vi "Lift.vi"(0 "LiftLocation":T1(ring)) -> ()   [LabVIEW 2018]
uses:
  <vilib>/Rock Robotics/SystemInterfaces/DIO/FPGA_DIOChannel.ctl
  <vilib>/Rock Robotics/WPI/ThirdParty/Phoenix-LabVIEW/Motor Controller/Controls/CTRE_Phoenix_MotorControl_ControlMode.ctl
  Lift Global.vi
  Times/Times Global.vi
  <vilib>/addons/control/pid/pid.llb/PID (DBL).vi
  <vilib>/Rock Robotics/WPI/ThirdParty/Phoenix-LabVIEW/Motor Controller/Get/CTRE_Phoenix_MotorController_GetSelectedSensorData.vi
  Cargo Intake/Cargo Intake Global.vi
  <vilib>/addons/control/pid/NI_PID_pid.lvlib
  <vilib>/Rock Robotics/WPI/Counter/WPI_CounterDigitalInputToDigitalSource.vi
panel:
  in  "t":dbl=0.5 format="%#_13g"
  in  "output range":cluster{"output high":dbl, "output low":dbl}={"output high"=1.0, "output low"=-1.0}
  in  "LiftMode":T2(ring)=enum."Basic Control"
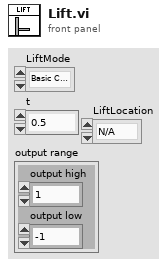
[diagram p1: front panel]
types:
  T1 = enum16{"N/A", "Hatch Panel Zone 1", "Hatch Panel Zone 2", "Hatch Panel Zone 3", "Cargo Zone 1", "Cargo Zone 2", "Cargo Zone 3"}
  T2 = enum16{"Ultra Manual Control", "Manual Control", "Basic Control", "Automated Control", "Autonomous Control"}
  T3 = typedef "FPGA_DIOChannel.ctl" = enum8{"DIO 0", "DIO 1", "DIO 2", "DIO 3", "DIO 4", "DIO 5", "DIO 6", "DIO 7", "DIO 8", "DIO 9", "DIO MXP 0", "DIO MXP 1", "DIO MXP 2", "DIO MXP 3", "DIO MXP 4", "DIO MXP 5", "DIO MXP 6", "DIO MXP 7", "DIO MXP 8", "DIO MXP 9", "DIO MXP 10", "DIO MXP 11", "DIO MXP 12", "DIO MXP 13", "DIO MXP 14", "DIO MXP 15", "SPI Port CS1", "SPI Port CS2", "SPI Port CS3", "SPI Port MISO", "SPI Port MOSI", "Invalid"}
  T4 = typedef "WPI_DigitalInputDevRef.ctl" = cluster{"DevStatus":errorcluster, "DIO Channel":T3}
  T5 = typedef "FPGA_CounterEncoderSourceConvertionLVSourceType.ctl" = cluster{"DevStatus":errorcluster, "AnalogTriggerMode?":bool, "DigitalMode":cluster{"DIO Channel":T6}, "AnalogTriggerMode":cluster{"AnalogTriggerIndex":T7, "OutputType":T8}}
  T6 = typedef "FPGA_DIODigitalSourceChannel.ctl" = enum8{"DIO 0", "DIO 1", "DIO 2", "DIO 3", "DIO 4", "DIO 5", "DIO 6", "DIO 7", "DIO 8", "DIO 9", "DIO MXP 0", "DIO MXP 1", "DIO MXP 2", "DIO MXP 3", "DIO MXP 4", "DIO MXP 5", "DIO MXP 6", "DIO MXP 7", "DIO MXP 8", "DIO MXP 9", "DIO MXP 10", "DIO MXP 11", "DIO MXP 12", "DIO MXP 13", "DIO MXP 14", "DIO MXP 15", "SPI Port CS1", "SPI Port CS2", "SPI Port CS3", "SPI Port MISO", "SPI Port MOSI", "Disabled"}
  T7 = typedef "FPGA_AnalogTriggerIndex.ctl" = enum8{"Trig 0", "Trig 1", "Trig 2", "Trig 3", "Trig 4", "Trig 5", "Trig 6", "Trig 7", "Invalid"}
  T8 = typedef "FPGA_AnalogTriggerOutType.ctl" = enum16{"InWindow", "TriggerState", "Rising", "Falling"}
  T9 = typedef "WPI_EncoderDevRef.ctl" = cluster{"DevStatus":errorcluster, "EncoderIndex":T10, "CounterIndex":T11, "DistancePerCount":dbl, "Decoding Type":T12}
  T10 = typedef "FPGA_EncoderIdx.ctl" = enum8{"Enc 0", "Enc 1", "Enc 2", "Enc 3", "Enc 4", "Enc 5", "Enc 6", "Enc 7", "Invalid"}
  T11 = typedef "FPGA_CounterCtrSystemIndex.ctl" = enum8{"Ctr 0", "Ctr 1", "Ctr 2", "Ctr 3", "Ctr 4", "Ctr 5", "Ctr 6", "Ctr 7", "Invalid"}
  T12 = typedef "WPI_EncoderType.ctl" = enum16{"1x", "2x", "4x"}
  T13 = typedef "WPI_MotorControlDeviceRef.ctl" = cluster{"DeviceStatus":errorcluster, "Type":T14, "PWM":cluster{"PWM Channel":T15, "DeadBand":T16}, "CAN":cluster{"Device Number":u8, "SetOutput VI Ref":variant, "GetOutput VI Ref":variant, "Enable VI Ref":variant, "Disable VI Ref":variant, "Data":variant}, "Invert":bool, "DIO PWM":cluster{"PWM \"Enable\" Channel":T15, "DIOChannel":T3, "PWM Rate":dbl}}
  T14 = typedef "WPI_MotorControlType.ctl" = enum16{"PWM", "CAN", "DIO PWM"}
  T15 = typedef "FPGA_DIOPWMChannel.ctl" = enum8{"PWM 0", "PWM 1", "PWM 2", "PWM 3", "PWM 4", "PWM 5", "PWM 6", "PWM 7", "PWM 8", "PWM 9", "PWM MXP 0", "PWM MXP 1", "PWM MXP 2", "PWM MXP 3", "PWM MXP 4", "PWM MXP 5", "PWM MXP 6", "PWM MXP 7", "PWM MXP 8", "PWM MXP 9", "Invalid"}
  T16 = typedef "WPI_PWMDeadband.ctl" = cluster{"Name":string, "maxPositivePwm":i32, "minPositivePwm":i32, "centerPwm":i32, "maxNegativePwm":i32, "minNegativePwm":i32, "angularRange":u16}
  T17 = typedef "CTRE_Phoenix_MotorControl_ControlMode.ctl" = u16
  T18 = typedef "Control 3.ctl" = dbl
  T19 = cluster{"proportional gain (Kc)":dbl, "integral time(Ti, min)":dbl, "derivative time(Td, min) 2":dbl}
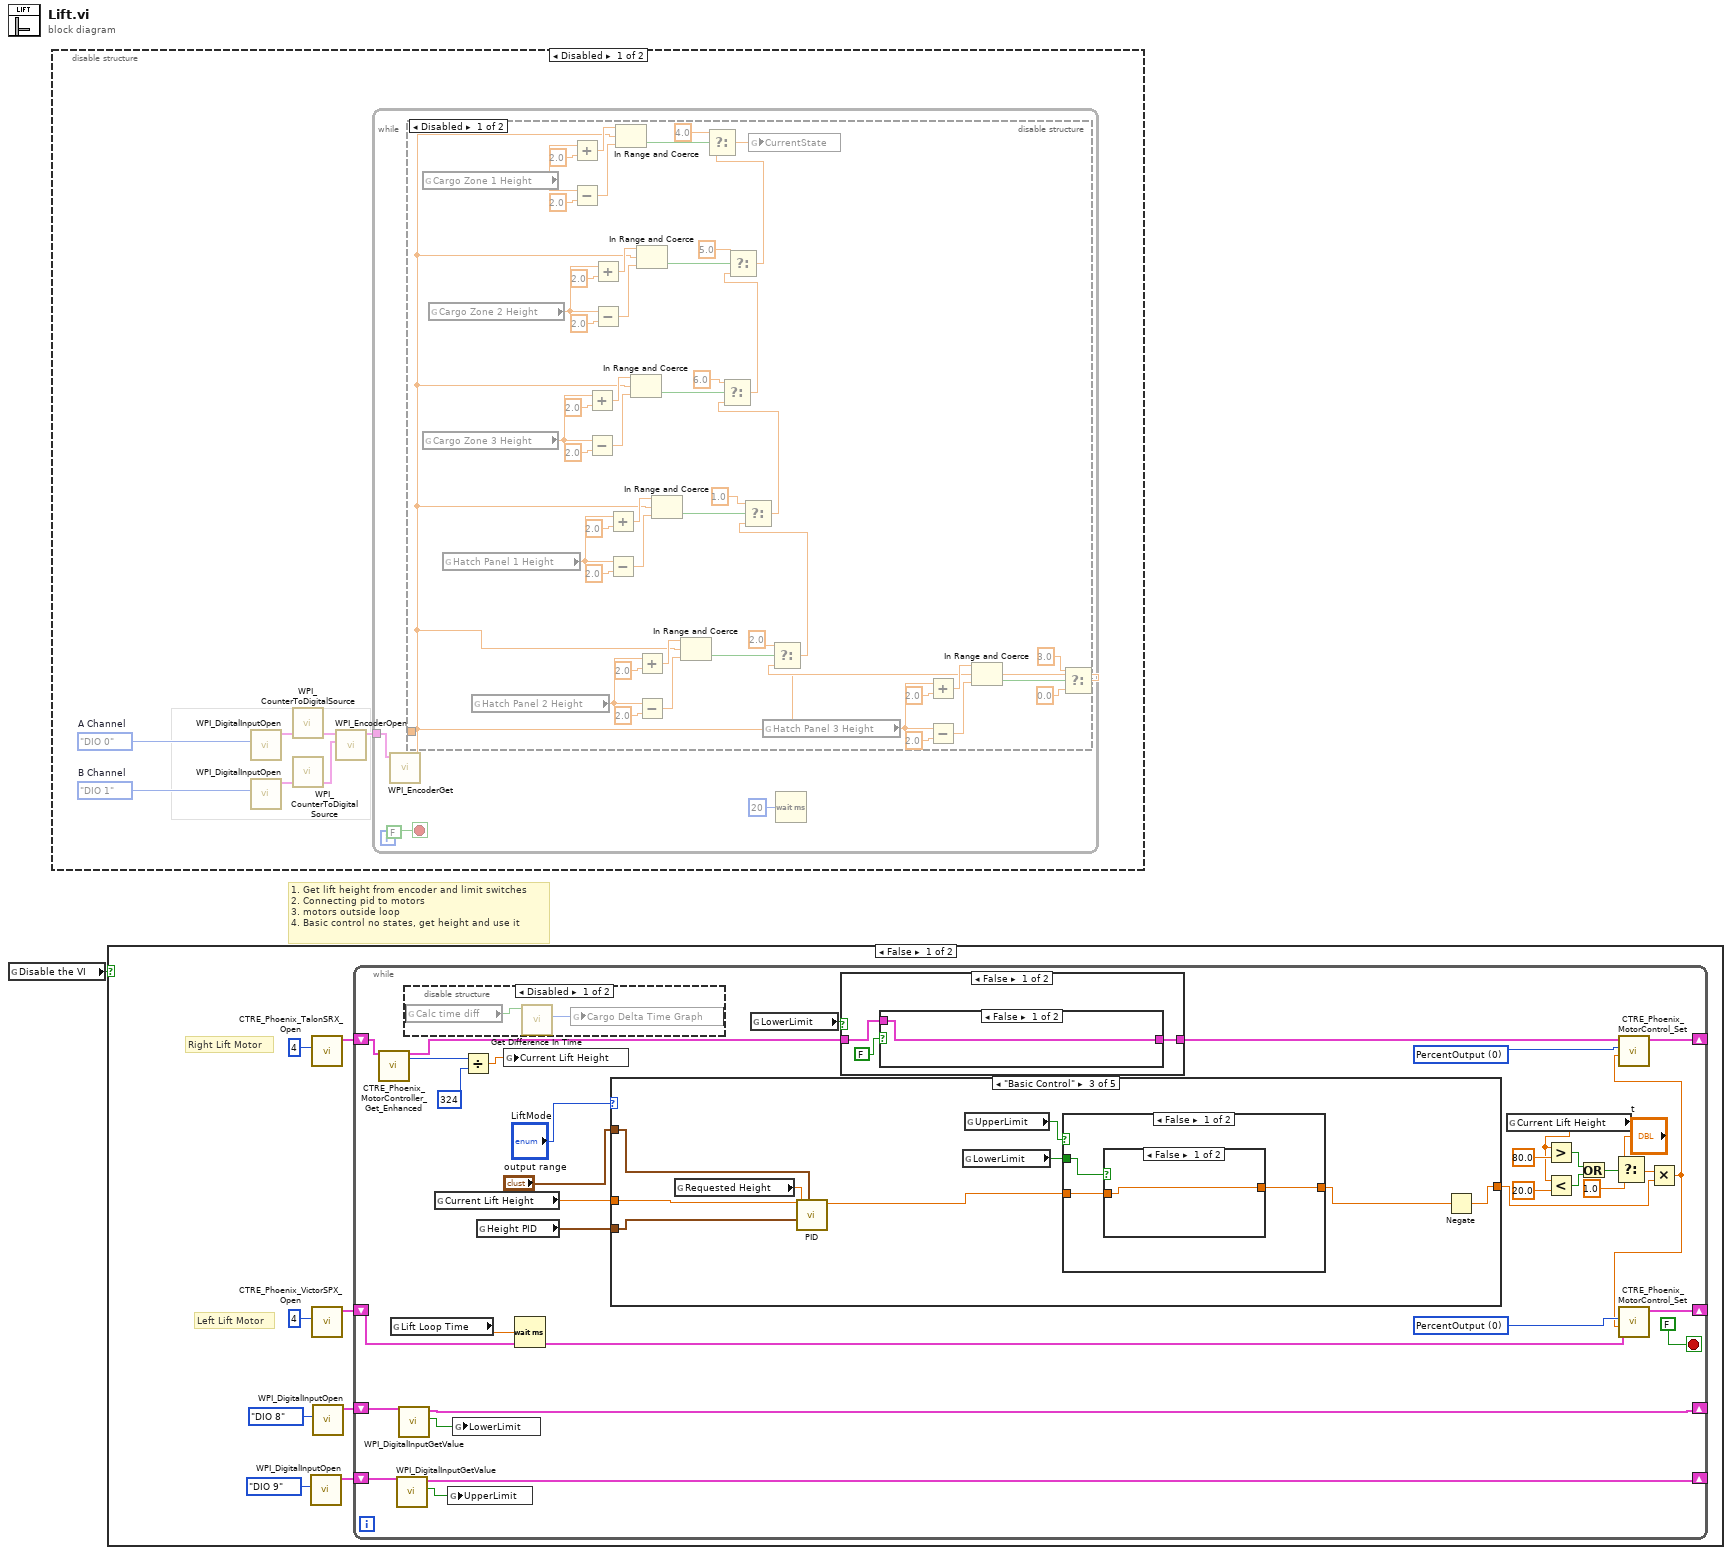
[diagram p0: block diagram]
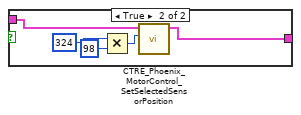
[diagram p4: hidden frame]
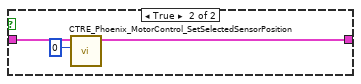
[diagram p5: hidden frame]
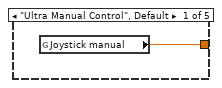
[diagram p7: hidden frame]
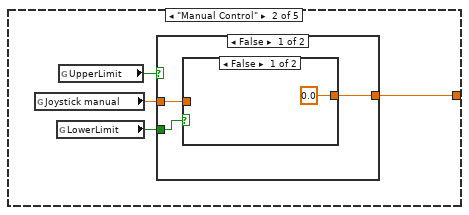
[diagram p8: hidden frame]
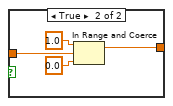
[diagram p9: hidden frame]
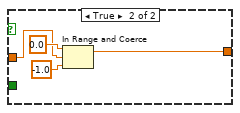
[diagram p10: hidden frame]
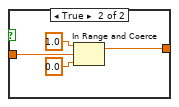
[diagram p11: hidden frame]
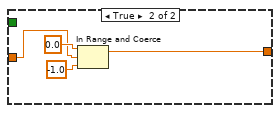
[diagram p12: hidden frame]
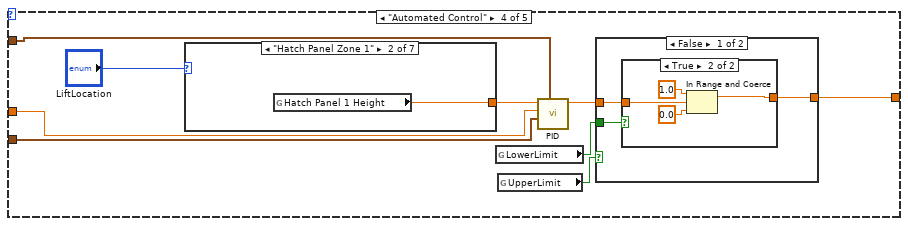
[diagram p13: hidden frame]
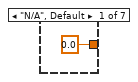
[diagram p14: hidden frame]
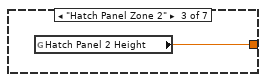
[diagram p15: hidden frame]
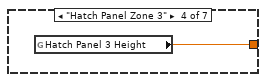
[diagram p16: hidden frame]
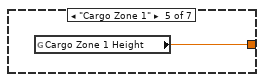
[diagram p17: hidden frame]
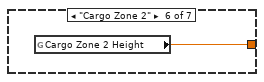
[diagram p18: hidden frame]
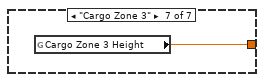
[diagram p19: hidden frame]
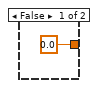
[diagram p20: hidden frame]
diagram:
  # "1. Get lift height from encoder and limit switches\n2. Connecting pid to motors\n3. motors outside loop\n4. Basic control no states, get height and use it"
  n1 = global read "Lift Global.vi" "Disable the VI"() -> (w1:bool)
  n2 = disable-structure shown="Disabled" {
    frame Disabled {
      w8 = FPGA_DIOChannel."DIO 1"  # B Channel
      w7 = FPGA_DIOChannel."DIO 0"  # A Channel
      n3 = call <vilib>:"WPI_DigitalInputOpen.vi"("DIO Channel"=w7) -> ("DigitalInputDevRef"=w4:T4)  [unwired: 1 in, 9 out]
      n4 = call <vilib>:"WPI_DigitalInputOpen.vi"("DIO Channel"=w8) -> ("DigitalInputDevRef"=w5:T4)  [unwired: 1 in, 9 out]
      n5 = call-poly <vilib>:"WPI_CounterToDigitalSource.vi"("DigitalInputDevRef"=w4) -> ("Digital Source"=w3:T5)  [unwired: 6 out]
      n6 = call-poly <vilib>:"WPI_CounterToDigitalSource.vi"("DigitalInputDevRef"=w5) -> ("Digital Source"=w6:T5)  [unwired: 6 out]
      n7 = call <vilib>:"WPI_EncoderOpen.vi"("BSource"=w6, "ASource"=w3) -> ("EncoderDevRef"=w2:T9)  [unwired: 6 in, 3 out]
      n8 = while {
        tunnel: w2 -> [w12]
        stop <- FALSE stop-if-true
        n9 = call <vilib>:"WPI_EncoderGet.vi"("EncoderDevRef"=w12) -> ("Distance"=w10:dbl)  [unwired: 5 in, 5 out]
        n10 = disable-structure shown="Disabled" {
          disable-tunnel: w10 -> [w13 _]
          frame Disabled {
            n11 = global read "Lift Global.vi" "Cargo Zone 1 Height"() -> (w53:dbl)
            n12 = global read "Lift Global.vi" "Cargo Zone 3 Height"() -> (w41:dbl)
            n13 = global read "Lift Global.vi" "Cargo Zone 2 Height"() -> (w59:dbl)
            n14 = global read "Lift Global.vi" "Hatch Panel 1 Height"() -> (w47:dbl)
            n15 = global read "Lift Global.vi" "Hatch Panel 2 Height"() -> (w29:dbl)
            n16 = Add(x=w53, y=2.0) -> (x+y=w55:dbl)
            n17 = Subtract(x=w53, y=2.0) -> (x-y=w56:dbl)
            n18 = Add(x=w41, y=2.0) -> (x+y=w43:dbl)
            n19 = Subtract(x=w41, y=2.0) -> (x-y=w44:dbl)
            n20 = Add(x=w59, y=2.0) -> (x+y=w61:dbl)
            n21 = Subtract(x=w59, y=2.0) -> (x-y=w62:dbl)
            n22 = Add(x=w47, y=2.0) -> (x+y=w49:dbl)
            n23 = Subtract(x=w47, y=2.0) -> (x-y=w50:dbl)
            n24 = In Range and Coerce(upper limit=w55, x=w13, lower limit=w56) -> (In Range?=w51:bool)  [unwired: 1 out]
            n25 = In Range and Coerce(upper limit=w43, x=w13, lower limit=w44) -> (In Range?=w39:bool)  [unwired: 1 out]
            n26 = In Range and Coerce(upper limit=w61, x=w13, lower limit=w62) -> (In Range?=w57:bool)  [unwired: 1 out]
            n27 = Add(x=w29, y=2.0) -> (x+y=w31:dbl)
            n28 = Subtract(x=w29, y=2.0) -> (x-y=w32:dbl)
            n29 = In Range and Coerce(upper limit=w49, x=w13, lower limit=w50) -> (In Range?=w45:bool)  [unwired: 1 out]
            n30 = In Range and Coerce(upper limit=w31, x=w13, lower limit=w32) -> (In Range?=w27:bool)  [unwired: 1 out]
            n31 = global read "Lift Global.vi" "Hatch Panel 3 Height"() -> (w35:dbl)
            n32 = Add(x=w35, y=2.0) -> (x+y=w37:dbl)
            n33 = Subtract(x=w35, y=2.0) -> (x-y=w38:dbl)
            n34 = In Range and Coerce(upper limit=w37, x=w13, lower limit=w38) -> (In Range?=w33:bool)  [unwired: 1 out]
            n35 = Select(t=3.0, s=w33, f=0.0 ("t")) -> (s? t:f=w23:dbl)
            n36 = Select(t=2.0, s=w27, f=w23) -> (s? t:f=w24:dbl)
            n37 = Select(t=1.0, s=w45, f=w24) -> (s? t:f=w25:dbl)
            n38 = Select(t=6.0, s=w39, f=w25) -> (s? t:f=w26:dbl)
            n39 = Select(t=5.0, s=w57, f=w26) -> (s? t:f=w20:dbl)
            n40 = Select(t=4.0, s=w51, f=w20) -> (s? t:f=w21:dbl)
            n41 = global write "Lift Global.vi" "CurrentState"(w21) -> ()
          }
          frame Enabled {
          }
        }
        n42 = Wait (ms)(milliseconds to wait=u32 20) -> ()  [unwired: 1 out]
      }
    }
    frame Enabled {
    }
  }
  n43 = case shown="False" w1 {
    frame False {
      # "Left Lift Motor"
      # "Right Lift Motor"
      n44 = call <vilib>:"WPI_DigitalInputOpen.vi"("DIO Channel"=FPGA_DIOChannel."DIO 9") -> ("DigitalInputDevRef"=w63:T4)  [unwired: 9 in, 1 out]
      n45 = call <vilib>:"CTRE_Phoenix_TalonSRX_Open.vi"("Device Number"=u8 4) -> ("CAN Talon SRX Ref"=w70:T13)  [unwired: 9 in, 1 out]
      n46 = call <vilib>:"CTRE_Phoenix_VictorSPX_Open.vi"("Device Number"=u8 4) -> ("CAN Talon SRX Ref"=w68:T13)  [unwired: 9 in, 1 out]
      n47 = call <vilib>:"WPI_DigitalInputOpen.vi"("DIO Channel"=FPGA_DIOChannel."DIO 8") -> ("DigitalInputDevRef"=w65:T4)  [unwired: 9 in, 1 out]
      n48 = while {
        shift-right: [w101] -> _
        shift-left: w70 -> [w94]
        shift-right: [w99] -> _
        shift-left: w68 -> [w98]
        shift-right: [w87] -> _
        shift-left: w65 -> [w88]
        shift-right: [w82] -> _
        shift-left: w63 -> [w83]
        stop <- FALSE stop-if-true
        w100 = T17 0 items=["PercentOutput"=0, "Position"=1, "Velocity"=2, "Current"=3, "Follower"=5, "MotionProfile"=6, "MotionMagic"=7, "MotionProfileArc"=10, "Disabled"=15] ("Control Mode")
        w102 = T17 0 items=["PercentOutput"=0, "Position"=1, "Velocity"=2, "Current"=3, "Follower"=5, "MotionProfile"=6, "MotionMagic"=7, "MotionProfileArc"=10, "Disabled"=15] ("Control Mode")
        n49 = call-poly <vilib>:"CTRE_Phoenix_MotorController_Get_Enhanced.vi"("PhoenixMotorControlDevRef"=w94) -> ("PhoenixMotorControlDevRef"=w93:T13, "Position (Raw Sensor Units)"=w91:i32)  [unwired: 11 in, 2 out]
        n50 = global read "Times Global.vi" "Lift Loop Time"() -> (w105:T18)
        n51 = call <vilib>:"WPI_DigitalInputGetValue.vi"("DigitalInputDevRef"=w83) -> ("Value"=w85:bool, "DigitalInputDevRef"=w82:T4)  [unwired: 8 in, 1 out]
        n52 = call <vilib>:"WPI_DigitalInputGetValue.vi"("DigitalInputDevRef"=w88) -> ("Value"=w86:bool, "DigitalInputDevRef"=w87:T4)  [unwired: 8 in, 1 out]
        n53 = disable-structure shown="Disabled" {
          frame Disabled {
            n54 = global read "Cargo Intake Global.vi" "Calc time diff"() -> (w119:bool)
            n55 = call "Get Difference In Time.vi"("Calculate Time Difference"=w119) -> ("Delta Time over Time"=w118:u32)  [unwired: 9 in, 1 out]
            n56 = global write "Times Global.vi" "Cargo Delta Time Graph"(w118) -> ()
          }
          frame Enabled {
          }
        }
        n57 = global read "Lift Global.vi" "Current Lift Height"() -> (w95:dbl)
        n58 = global write "Lift Global.vi" "UpperLimit"(w85) -> ()
        n59 = global write "Lift Global.vi" "LowerLimit"(w86) -> ()
        n60 = Divide(x=w91, y=324) -> (x/y=w90:dbl)
        n61 = global read "Lift Global.vi" "Height PID"() -> (w96:T19)
        n62 = global write "Lift Global.vi" "Current Lift Height"(w90) -> ()
        n63 = Wait (ms)(milliseconds to wait=w105) -> ()  [unwired: 1 out]
        n64 = case shown="\"Basic Control\"" "LiftMode" {
          tunnel: [w120 w121 w141 w163 0.0 ("Cargo Zone 3 Height")] -> w74
          tunnel: w95 -> [_ _ w145 w161 _]
          tunnel: w96 -> [_ _ w144 w160 _]
          tunnel: "output range" -> [_ _ w143 w162 _]
          frame "Ultra Manual Control", Default {
            n65 = global read "Lift Global.vi" "Joystick manual"() -> (w120:dbl)
          }
          frame "Manual Control" {
            n66 = global read "Lift Global.vi" "Joystick manual"() -> (w122:dbl)
            n67 = global read "Lift Global.vi" "LowerLimit"() -> (w124:bool)
            n68 = global read "Lift Global.vi" "UpperLimit"() -> (w123:bool)
            n69 = case shown="False" w123 {
              tunnel: w124 -> [w127 _]
              tunnel: [w126 w134] -> w121
              tunnel: w122 -> [w125 w133]
              frame False {
                n70 = case shown="False" w127 {
                  tunnel: [0.0 w132] -> w126
                  tunnel: w125 -> [_ w129]
                  frame False {
                  }
                  frame True {
                    n71 = In Range and Coerce(upper limit=1.0, x=w129, lower limit=0.0) -> (coerced(x)=w132:dbl)  [unwired: 1 out]
                  }
                }
              }
              frame True {
                n72 = In Range and Coerce(upper limit=0.0, x=w133, lower limit=-1.0) -> (coerced(x)=w134:dbl)  [unwired: 1 out]
              }
            }
          }
          frame "Basic Control" {
            n73 = global read "Lift Global.vi" "Requested Height"() -> (w142:dbl)
            n74 = call-poly <vilib>:"PID.vi"("output range"=w143, "PID gains"=w144, "process variable"=w145, "setpoint"=w142) -> ("output"=w138:dbl)  [unwired: 6 in, 1 out]
            n75 = global read "Lift Global.vi" "LowerLimit"() -> (w140:bool)
            n76 = global read "Lift Global.vi" "UpperLimit"() -> (w139:bool)
            n77 = case shown="False" w139 {
              tunnel: w140 -> [w148 _]
              tunnel: [w147 w155] -> w137
              tunnel: w138 -> [w146 w154]
              frame False {
                n78 = case shown="False" w148 {
                  tunnel: [w149 w153] -> w147
                  tunnel: w146 -> [w149 w150]
                  frame False {
                  }
                  frame True {
                    n79 = In Range and Coerce(upper limit=1.0, x=w150, lower limit=0.0) -> (coerced(x)=w153:dbl)  [unwired: 1 out]
                  }
                }
              }
              frame True {
                n80 = In Range and Coerce(upper limit=0.0, x=w154, lower limit=-1.0) -> (coerced(x)=w155:dbl)  [unwired: 1 out]
              }
            }
            n81 = Negate(x=w137) -> (-x=w141:dbl)
          }
          frame "Automated Control" {
            n82 = case shown="\"Hatch Panel Zone 1\"" "LiftLocation" {
              tunnel: [0.0 ("Cargo Zone 3 Height") w168 w169 w170 w171 w172 w173] -> w158
              frame "N/A", Default {
              }
              frame "Hatch Panel Zone 1" {
                n83 = global read "Lift Global.vi" "Hatch Panel 1 Height"() -> (w168:dbl)
              }
              frame "Hatch Panel Zone 2" {
                n84 = global read "Lift Global.vi" "Hatch Panel 2 Height"() -> (w169:dbl)
              }
              frame "Hatch Panel Zone 3" {
                n85 = global read "Lift Global.vi" "Hatch Panel 3 Height"() -> (w170:dbl)
              }
              frame "Cargo Zone 1" {
                n86 = global read "Lift Global.vi" "Cargo Zone 1 Height"() -> (w171:dbl)
              }
              frame "Cargo Zone 2" {
                n87 = global read "Lift Global.vi" "Cargo Zone 2 Height"() -> (w172:dbl)
              }
              frame "Cargo Zone 3" {
                n88 = global read "Lift Global.vi" "Cargo Zone 3 Height"() -> (w173:dbl)
              }
            }
            n89 = global read "Lift Global.vi" "LowerLimit"() -> (w166:bool)
            n90 = global read "Lift Global.vi" "UpperLimit"() -> (w165:bool)
            n91 = call-poly <vilib>:"PID.vi"("output range"=w162, "PID gains"=w160, "process variable"=w161, "setpoint"=w158) -> ("output"=w164:dbl)  [unwired: 6 in, 1 out]
            n92 = case shown="False" w165 {
              tunnel: w166 -> [w176 _]
              tunnel: [w175 w183] -> w163
              tunnel: w164 -> [w174 w182]
              frame False {
                n93 = case shown="True" w176 {
                  tunnel: [0.0 w181] -> w175
                  tunnel: w174 -> [_ w178]
                  frame False {
                  }
                  frame True {
                    n94 = In Range and Coerce(upper limit=1.0, x=w178, lower limit=0.0) -> (coerced(x)=w181:dbl)  [unwired: 1 out]
                  }
                }
              }
              frame True {
                n95 = In Range and Coerce(upper limit=0.0, x=w182, lower limit=-1.0) -> (coerced(x)=w183:dbl)  [unwired: 1 out]
              }
            }
          }
          frame "Autonomous Control" {
          }
        }
        n96 = global read "Lift Global.vi" "LowerLimit"() -> (w84:bool)
        n97 = case shown="False" w84 {
          tunnel: w93 -> [w108 w117]
          tunnel: [w107 w116] -> w92
          frame False {
            n98 = case shown="False" FALSE {
              tunnel: w108 -> [w109 w114]
              tunnel: [w109 w113] -> w107
              frame False {
              }
              frame True {
                n99 = Multiply(x=324 ("y"), y=98 ("New Sensor Position")) -> (x*y=w110:i32)
                n100 = call <vilib>:"CTRE_Phoenix_MotorControl_SetSelectedSensorPosition.vi"("New Sensor Position"=w110, "PhoenixMotorControlDevRef"=w114) -> ("PhoenixMotorControlDevRef"=w113:T13)  [unwired: 8 in, 1 out]
              }
            }
          }
          frame True {
            n101 = call <vilib>:"CTRE_Phoenix_MotorControl_SetSelectedSensorPosition.vi"("New Sensor Position"=0, "PhoenixMotorControlDevRef"=w117) -> ("PhoenixMotorControlDevRef"=w116:T13)  [unwired: 8 in, 1 out]
          }
        }
        n102 = global read "Lift Global.vi" "Current Lift Height"() -> (w79:dbl)
        n103 = Greater?(x=w79, y=80.0) -> (0:w77:bool)
        n104 = Less?(x=w79, y=20.0) -> (x < y?=w78:bool)
        n105 = Or(x=w77, y=w78) -> (x .or. y?=w76:bool)
        n106 = Select(t="t", s=w76, f=1.0) -> (s? t:f=w75:dbl)
        n107 = Multiply(x=w75, y=w74) -> (x*y=w71:dbl)
        n108 = call <vilib>:"CTRE_Phoenix_MotorControl_Set.vi"("Output"=w71, "Control Mode"=w102, "PhoenixMotorControlDevRef"=w92) -> ("PhoenixMotorControlDevRef"=w101:T13)  [unwired: 7 in, 1 out]
        n109 = call <vilib>:"CTRE_Phoenix_MotorControl_Set.vi"("Output"=w71, "Control Mode"=w100, "PhoenixMotorControlDevRef"=w98) -> ("PhoenixMotorControlDevRef"=w99:T13)  [unwired: 7 in, 1 out]
      }
    }
    frame True {
    }
  }
